vi "PH_DataViewer.contents.vi"   [LabVIEW 2014, in "PH_DataViewer.lvlib"]
doc: "This class is forseen to inspect shot data. Several of them can be saved in ASCI format.\n\nThis class is part of the PHELIX user layer."
uses:
  PH_DataViewer.lvlib
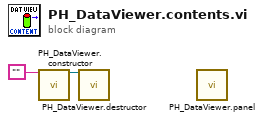
[diagram p0: block diagram]
diagram:
  n1 = call "PH_DataViewer.constructor.vi"("name"="") -> ("i ref out"=w2:refnum<vi>)  [unwired: 16 in, 2 out]
  n2 = call "PH_DataViewer.destructor.vi"("i ref in"=w2) -> ()  [unwired: 18 in, 1 out]
  n3 = call "PH_DataViewer.panel.vi"() -> ()  [unwired: 19 in, 1 out]
